vi "absorption_cross_section.vi"(8 "Linewidth (MHz)":dbl, 9 "Detuning (MHz)":dbl, 10 "Wavelength (m)":dbl) -> (2 "Cross Section (um^2)":dbl)   [LabVIEW 2016]
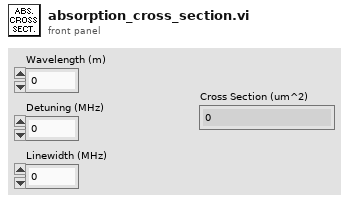
[diagram p1: front panel]
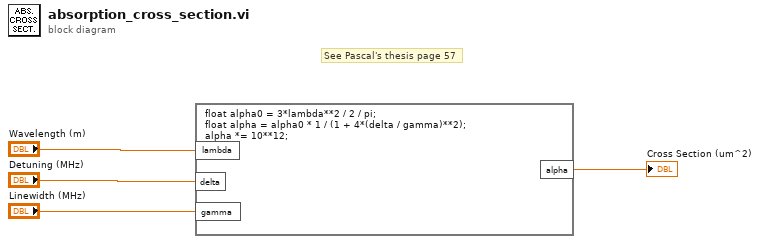
[diagram p0: block diagram]
diagram:
  # "See Pascal's thesis page 57"
  n1 = formula code="float alpha0 = 3*lambda**2 / 2 / pi;\nfloat alpha = alpha0 * 1 / (1 + 4*(delta / gamma)**2);\nalpha *= 10**12;"("lambda"="Wavelength (m)", "delta"="Detuning (MHz)", "gamma"="Linewidth (MHz)") -> ("alpha"=→"Cross Section (um^2)":dbl)
